vi "Make Dlg Modal at Runtime.vi"(4 "error in (no error)":errorcluster, 6 "Action":T1) -> (0 "error out":errorcluster)   [LabVIEW 2013, in "Utilities 1.lvlib"]
doc: "Two Modes:\nOpen Dialog - Make all the IMAQ windows non floating before making the calling vi visible\nClose Dialog - Make the calling vi non visible then make the IMAQ window floating\n\nIf the input path is empty then the floating of the IMAQ window is handled but the showing or hiding of the calling vi is not performed."
uses:
  Utilities 1.lvlib
  Controls/Make Dialog Action Enum.ctl
  Make Modal Global.vi
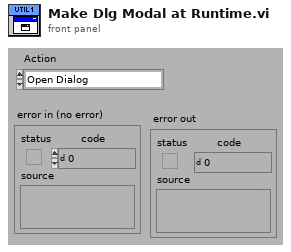
[diagram p1: front panel]
types:
  T1 = typedef "Utilities 1.lvlib/Make Dialog Action Enum.ctl" = enum16{"Open Dialog", "Open Frontmost", "Close Dialog"}
  T2 = enum32{"Invalid", "Standard", "Closed", "Hidden", "Minimized", "Maximized"}
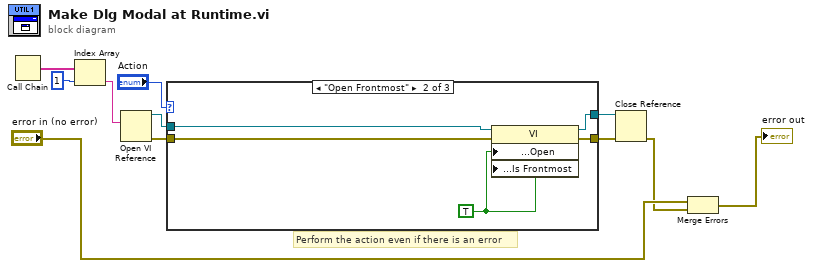
[diagram p0: block diagram]
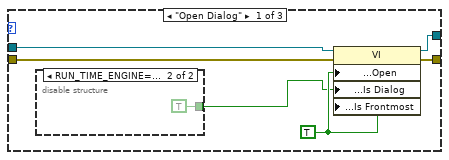
[diagram p2: hidden frame]
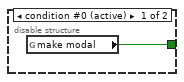
[diagram p3: hidden frame]
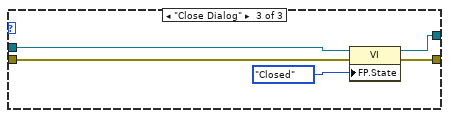
[diagram p4: hidden frame]
diagram:
  # "Perform the action even if there is an error"
  n1 = Call Chain() -> (call chain=w10:string[])
  n2 = Index Array(array=w10, index=1) -> (element=w8:string)
  n3 = Open VI Reference(vi path=w8) -> (vi reference=w1:refnum<vi>, error out=w5:errorcluster)  [unwired: 5 in]
  n4 = case shown="\"Open Frontmost\"" "Action" {
    tunnel: w1 -> [w16 w23 w28]
    tunnel: [w15 w22 w27] -> w7
    tunnel: [w13 w20 w26] -> w6
    tunnel: w5 -> [w14 w21 w25]
    frame "Open Dialog" {
      w17 = TRUE ("Front Panel Window:Open")
      n5 = disable-structure shown="RUN_TIME_ENGINE==True" {
        disable-tunnel: [w18 TRUE ("make modal")] -> w12
        frame condition #0 (active) {
          n6 = global read "Make Modal Global.vi" "make modal"() -> (w18:bool)
        }
        frame condition #1 {
        }
      }
      n7 = property class="VI"(reference=w16, error in=w14, "Front Panel Window:Open"=w17, "Front Panel Window:Is Dialog"=w12, "Front Panel Window:Is Frontmost"=w17) -> (reference out=w15:refnum<vi>, error out=w13:errorcluster)
    }
    frame "Open Frontmost" {
      w24 = TRUE ("Front Panel Window:Open")
      n8 = property class="VI"(reference=w23, error in=w21, "Front Panel Window:Open"=w24, "Front Panel Window:Is Frontmost"=w24) -> (reference out=w22:refnum<vi>, error out=w20:errorcluster)
    }
    frame "Close Dialog" {
      n9 = property class="VI"(reference=w28, error in=w25, "FP.State"=T2."Closed" ("Front Panel Window:State")) -> (reference out=w27:refnum<vi>, error out=w26:errorcluster)
    }
  }
  n10 = Close Reference(reference=w7, error in (no error)=w6) -> (error out=w3:errorcluster)
  n11 = Merge Errors("error in (no error)", w3) -> (→"error out":errorcluster)
